vi "Get Queue Timeout.vi"(11 "SessionHandler in":refnum<class "SessionHandler.lvclass">) -> (3 "SessionHandler out":refnum<class "SessionHandler.lvclass">, 4 "Queue Timeout":i32)   [LabVIEW 2019, in "Network Sink.lvlib" / "SessionHandler.lvclass"]
uses:
  <vilib>/gpm_packages/@cs/event-logger/Source/Network Sink/SessionHandler/SessionHandler.lvclass
  <vilib>/gpm_packages/@cs/event-logger/Source/Network Sink/SessionHandler/SessionHandler.lvclass/SessionHandler.ctl
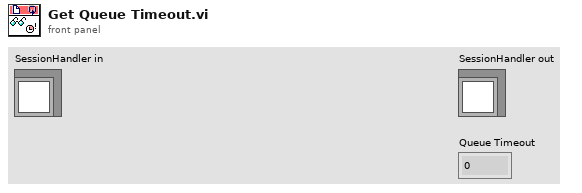
[diagram p1: front panel]
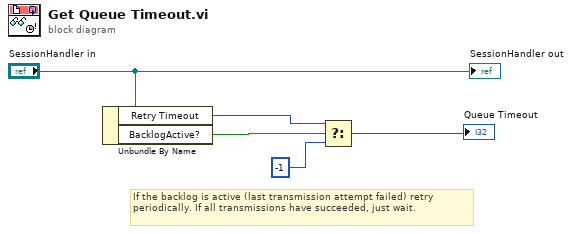
[diagram p0: block diagram]
diagram:
  # "If the backlog is active (last transmission attempt failed) retry periodically. If all transmissions have succeeded, just wait."
  n1 = Unbundle By Name("SessionHandler in") -> ("Retry Timeout"=w3:i32, "BacklogActive?"=w4:bool)
  n2 = Select(t=w3, s=w4, f=-1) -> (s? t:f=→"Queue Timeout":i32)
  "SessionHandler out" <- "SessionHandler in"
